vi "PH_IEEE1394Camera.contents.vi"   [LabVIEW 2014, in "PH_IEEE1394Camera.lvlib"]
doc: "This class controls a IEEE 1394 camera.\n\nThis class is part of the PHELIX user layer."
uses:
  PH_IEEE1394Camera.lvlib
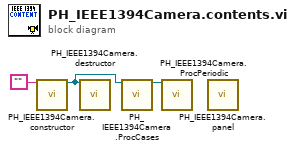
[diagram p0: block diagram]
diagram:
  n1 = call "PH_IEEE1394Camera.constructor.vi"("name"="") -> ("i ref out"=w1:refnum<vi>)  [unwired: 16 in, 2 out]
  n2 = call "PH_IEEE1394Camera.destructor.vi"("i ref in"=w1) -> ()  [unwired: 18 in, 1 out]
  n3 = call "PH_IEEE1394Camera.ProcCases.vi"("i ref in"=w1) -> ("i ref out"=w3:refnum<vi>)  [unwired: 16 in, 2 out]
  n4 = call "PH_IEEE1394Camera.ProcPeriodic.vi"("i ref in"=w3) -> ()  [unwired: 16 in, 3 out]
  n5 = call "PH_IEEE1394Camera.panel.vi"() -> ()  [unwired: 19 in, 1 out]
